vi "Begin-End Map.vi"(8 "Error In":errorcluster) -> (0 "Error Out":errorcluster)   [LabVIEW 2017, in "Tests.lvlib" / "Writer.lvlib"]
uses:
  Writer.lvlib
  src/LabPack/Public/Writer/Private/Begin Map by Value.vi
  src/LabPack/Public/Writer/Private/End Map by Value.vi
  <vilib>/addons/_JKI Toolkits/Caraya/classes/Test/Test.lvclass
  <vilib>/addons/_JKI Toolkits/Caraya/classes/Assert/Assert.lvclass
  src/LabPack/Public/Writer/Writer.lvclass
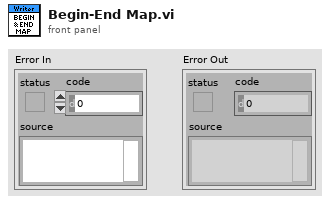
[diagram p1: front panel]
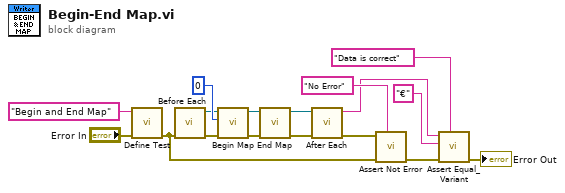
[diagram p0: block diagram]
diagram:
  n1 = call <vilib>:"Define Test.vi"("error in (no error)"="Error In", "Label (VI Title)"="Begin and End Map") -> ("error out"=w13:errorcluster)  [unwired: 9 in]
  n2 = call "Before Each.vi"("Error In"=w13) -> ("Error Out"=w4:errorcluster, "Writer Out"=w5:refnum<class "Writer.lvclass">)  [unwired: 9 in]
  n3 = call-poly "Begin Map.vi"("Error In"=w4, "Elements Count"=u32 0, "Writer In"=w5) -> ("Error Out"=w9:errorcluster, "Writer Out"=w12:refnum<class "Writer.lvclass">)  [unwired: 7 in]
  n4 = call-poly "End Map.vi"("Error In"=w9, "Writer In"=w12) -> ("Error Out"=w8:errorcluster, "Writer Out"=w10:refnum<class "Writer.lvclass">)  [unwired: 8 in]
  n5 = call "After Each.vi"("Error In"=w8, "Writer In"=w10) -> ("Error Out"=w2:errorcluster, "Data"=w3:string)  [unwired: 8 in]
  n6 = call <vilib>:"Assert Not Error.vi"("Label"="No Error", "error in (no error)"=w13, "Not Error?"=w2) -> ("error out"=w15:errorcluster)  [unwired: 8 in]
  n7 = call <vilib>:"Assert Equal_Variant.vi"("Label"="Data is correct", "error in (no error)"=w15, "Y"="€" ("Data"), "X"=w3) -> ("error out"=→"Error Out":errorcluster)  [unwired: 7 in]
